vi "Unravel Index.vi"(2 "shape":i32[](array[numeric]), 3 "Flat Index":i32) -> (0 "In Range?":bool, 1 "ND Index":i32[](array[numeric]))   [LabVIEW 2020, in "VIM Tools.lvlib"]
uses:
  VIM Tools.lvlib
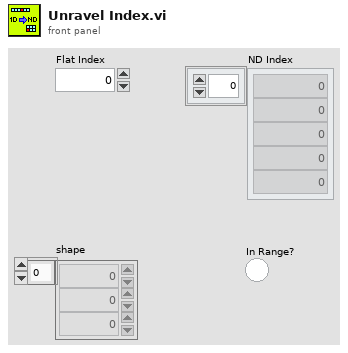
[diagram p1: front panel]
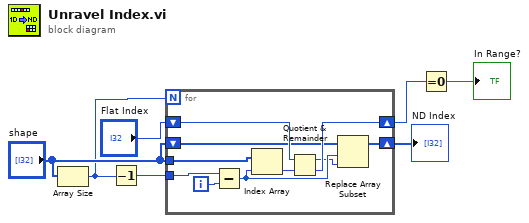
[diagram p0: block diagram]
diagram:
  n1 = Array Size(array="shape") -> (size(s)=w4:i32)
  n2 = Decrement(x=w4) -> (x-1=w3:i32)
  n3 = for {
    N: w4 -> [_]
    tunnel: "shape" -> [w15]
    shift-right: [w16] -> w2
    shift-left: "Flat Index" -> [w17]
    shift-right: [w12] -> w5
    shift-left: "shape" -> [w13]
    tunnel: w3 -> [w9]
    i -> [w8]
    n4 = Subtract(x=w9, y=w8) -> (x-y=w11:i32)
    n5 = Index Array(array=w15, index=w11) -> (element=w14:i32)
    n6 = Quotient & Remainder(x=w17, y=w14) -> (x-y*floor(x/y)=w10:i32, floor(x/y)=w16:i32)
    n7 = Replace Array Subset(array=w13, new element=w10, index=w11) -> (w12:i32[])
  }
  "ND Index" <- w5
  n8 = Equal To 0?(x=w2) -> (x = 0?=→"In Range?":bool)
